vi "Triangle.vi"(0 "error in":errorcluster, 5 "Amount of Points":i32, 7 "Amplitude":dbl, 9 "Duty Cycle":dbl=0.01 min=0.01 max=0.99, 11 "DC Offset":dbl) -> (4 "error out":errorcluster, 6 "Triangle wave array":dbl[](array[numeric]))   [LabVIEW 2020]
panel:
  out "x*y 2":dbl
  out "x*y":dbl
  out "Waveform Graph":dbl[](graph)
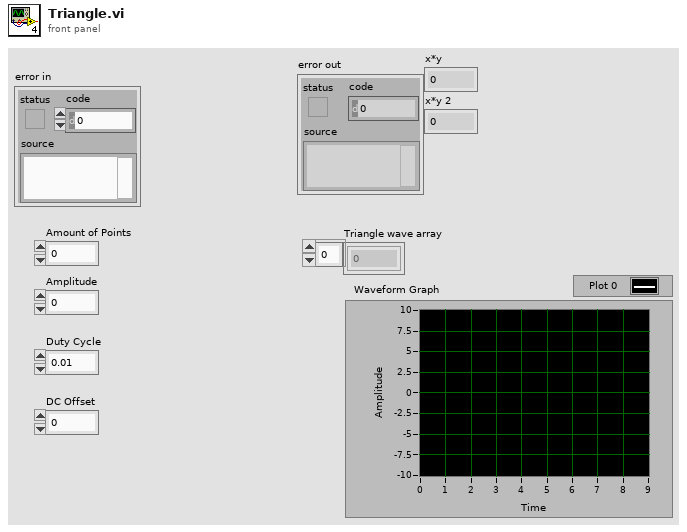
[diagram p1: front panel]
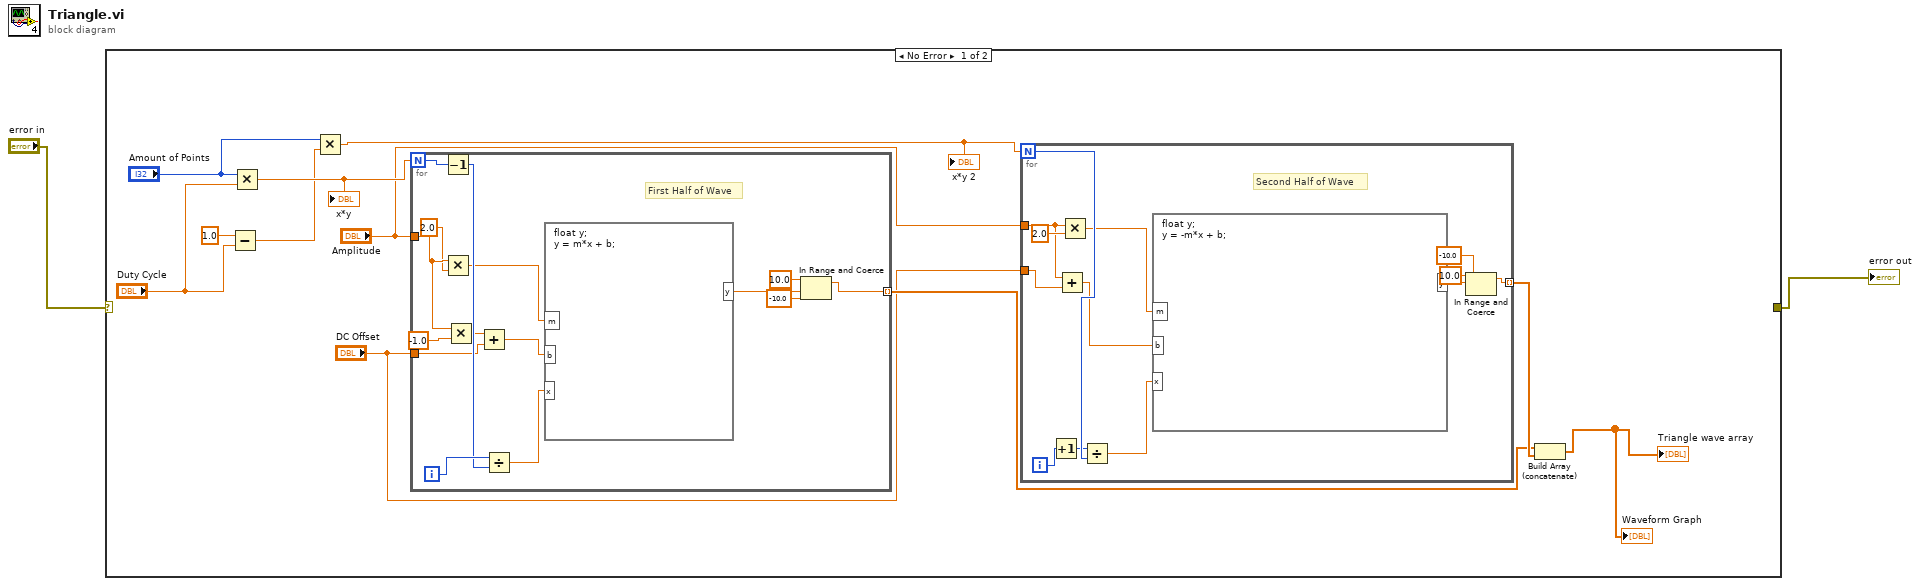
[diagram p0: block diagram]
diagram:
  n1 = case shown="No Error" "error in" {
    selector: "error in" -> [_ w42]
    tunnel: [_ w42] -> w1
    frame No Error {
      n2 = Subtract(x=1.0, y="Duty Cycle") -> (x-y=w9:dbl)
      n3 = Multiply(x="Amount of Points", y="Duty Cycle") -> (x*y=w12:dbl)
      "x*y" <- w12
      n4 = Multiply(x="Amount of Points", y=w9) -> (x*y=w7:dbl)
      "x*y 2" <- w7
      n5 = for {
        N: w12 -> [w40]
        tunnel: "Amplitude" -> [w33]
        tunnel: "DC Offset" -> [w35]
        tunnel: [w27] -> w6 mode=indexing
        i -> [w39]
        # "First Half of Wave"
        n6 = Decrement(x=w40) -> (x-1=w38:i32)
        n7 = Multiply(x=w33, y=2.0) -> (x*y=w31:dbl)
        n8 = Multiply(x=w33, y=-1.0) -> (x*y=w36:dbl)
        n9 = Add(x=w36, y=w35) -> (x+y=w34:dbl)
        n10 = Divide(x=w39, y=w38) -> (x/y=w41:dbl)
        n11 = formula code="float y;\ny = m*x + b;"("m"=w31, "x"=w41, "b"=w34) -> ("y"=w30:dbl)
        n12 = In Range and Coerce(upper limit=10.0, x=w30, lower limit=-10.0) -> (coerced(x)=w27:dbl)  [unwired: 1 out]
      }
      n13 = for {
        N: w7 -> [w24]
        tunnel: [w16] -> w13 mode=indexing
        tunnel: "Amplitude" -> [w20]
        tunnel: "DC Offset" -> [w21]
        i -> [w25]
        # "Second Half of Wave"
        n14 = Increment(x=w25) -> (x+1=w18:i32)
        n15 = Add(x=w20, y=w21) -> (x+y=w19:dbl)
        n16 = Multiply(x=w20, y=2.0) -> (x*y=w22:dbl)
        n17 = Divide(x=w18, y=w24) -> (x/y=w26:dbl)
        n18 = formula code="float y;\ny = -m*x + b;"("m"=w22, "x"=w26, "b"=w19) -> ("y"=w17:dbl)
        n19 = In Range and Coerce(upper limit=10.0, x=w17, lower limit=-10.0) -> (coerced(x)=w16:dbl)  [unwired: 1 out]
      }
      n20 = Build Array (concatenate)(w6, w13) -> (→"Triangle wave array" →"Waveform Graph":dbl[])
    }
    frame Error {
    }
  }
  "error out" <- w1
